vi "Example Custom LVClass Serialization.vi"() -> ()   [LabVIEW 2017]
uses:
  Demo LVClass Serializer.lvclass
  C:/Git/JSONtext/LVClass Serializer/JSONtext LVClass Serializer.lvclass
  <vilib>/drjdpowell/Messenging/Core Messages/Message/MSG.lvclass/MSG.ctl
  <vilib>/drjdpowell/Messenging/Core Messages/ObjectMessage/ObjectMSG.lvclass/ObjectMSG.ctl
  <vilib>/drjdpowell/Messenging/Core Messages/MSG Library/Write Message (Object).vi
  912a6c23-4bb1-4c3c-9308-e383c675d733.vi
  e1d0a090-eb0b-4084-98ba-e2f06df06374.vi
  <vilib>/drjdpowell/Messenging/Core Messages/Message/Overwrite Reply Address.vi
  <vilib>/drjdpowell/Messenging/Core Messages/ObjectMessage/Write ObjectMSG.vi
  <vilib>/drjdpowell/Messenging/Core Messages/Message/Label Message.vi
  <vilib>/drjdpowell/Messenging/Core Messages/ObjectMessage/ObjectMSG.lvclass
  C:/Program Files (x86)/National Instruments/LabVIEW 2017/vi.lib/drjdpowell/Messenging/Core Messages/Message/MSG.lvclass
  Variant to JSON Text.vi
  JSON text to Variant.vi
  <vilib>/drjdpowell/Messenging/Core Messengers/Send/Send.lvclass
  <vilib>/drjdpowell/Messenging/Core Messages/MSG Library/SendMSG.lvlib
  <vilib>/drjdpowell/Messenging/Core Messages/Message/MSG.lvclass
panel:
  out "Data out":T1
  out "x = y?":bool
  out "error out":errorcluster
  out "<JSON>":string
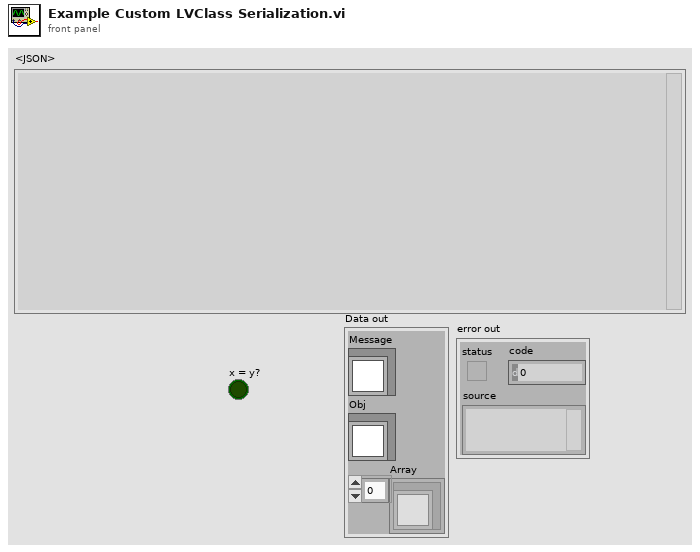
[diagram p1: front panel]
types:
  T1 = cluster{"Message":refnum<class>, "Obj":refnum<class>, "Array":refnum<class>[]}
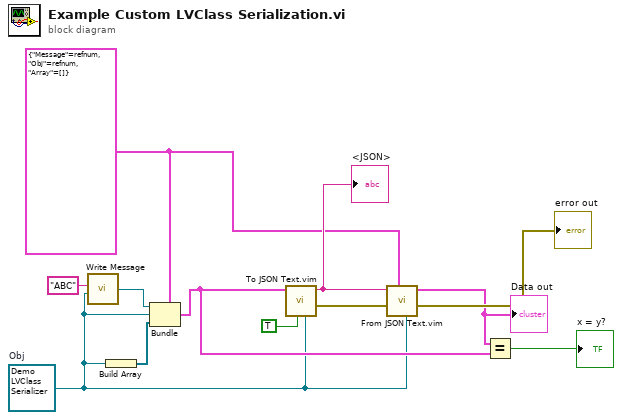
[diagram p0: block diagram]
diagram:
  w1 = T1 {"Message"=refnum, "Obj"=refnum, "Array"=[]} ("output cluster")
  w2 = refnum<class "Demo LVClass Serializer.lvclass"> refnum  # Obj
  n1 = call-poly <vilib>:"Write Message.vi"("Label"="ABC", "Contents"=w2) -> ("Message"=w6:refnum<class "MSG.lvclass">)  [unwired: 6 in]
  n2 = Build Array(w2) -> (w3:refnum<class "Demo LVClass Serializer.lvclass">[])
  n3 = Bundle(cluster=w1, "Message"=w6, "Obj"=w2, "Array"=w3) -> (w5:T1)
  n4 = call "To JSON Text.vim"("LVClass Serializer"=w2, "Pretty Print?"=TRUE, "Anything"=w5) -> ("error out"=w9:errorcluster, "<JSON>"=w10:string)  [unwired: 7 in]
  "<JSON>" <- w10
  n5 = call "From JSON Text.vim"("LVClass Serializer"=w2, "Data Type and Default Value"=w1, "error in (no error)"=w9, "JSON"=w10) -> ("error out"=→"error out":errorcluster, "Data out"=w4:T1)  [unwired: 6 in]
  "Data out" <- w4
  n6 = Equal?(x=w4, y=w5) -> (x = y?=→"x = y?":bool)
